vi "optionsAcq_channel_select.vi"(8 "error in (no error)":errorcluster, 9 "channelType_spectrum":T1, 10 "channel DUT (index)":i32, 11 "Thorlabs_OSA300_64 in":refnum<class "OSA300.lvclass">) -> (0 "error out":errorcluster, 2 "channel DUT out":i32, 3 "Thorlabs_OSA300_64 out":refnum<class "OSA300.lvclass">)   [LabVIEW 2010, in "OSA300.lvclass"]
doc: "Models within the OSA300/Redstone series typically have two detection channels, together they provide the total specified wavelength range. The channel index must be selected when acquiring interferograms, the default channel index is zero after init.vi. \n\nWhen acquiring a spectra, either the total wavelength range can be selected, (the ranges provided by all channels stiched together, referred to as a stiched spectra), or the range corresponding to one channel index.\n\nThe wavelength range associated with each channel can be read with instrumentProperties_channels.vi."
uses:
  OSA300.lvclass
  _misc/Thorlabs_FTS_misc.llb/channelType_spectrum.ctl
  OSA20X_misc.lvlib
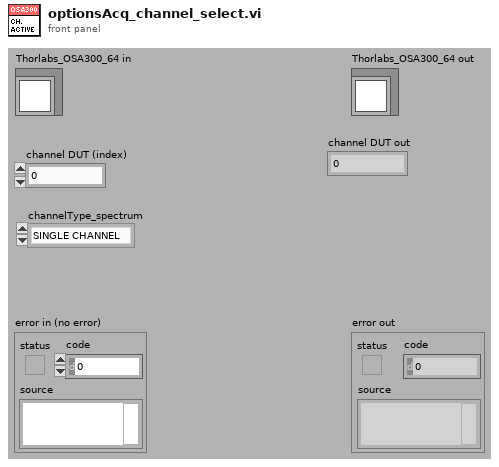
[diagram p1: front panel]
types:
  T1 = typedef "OSA20X_misc.lvlib/channelType_spectrum.ctl" = enum16{"SINGLE CHANNEL", "STICHED"}
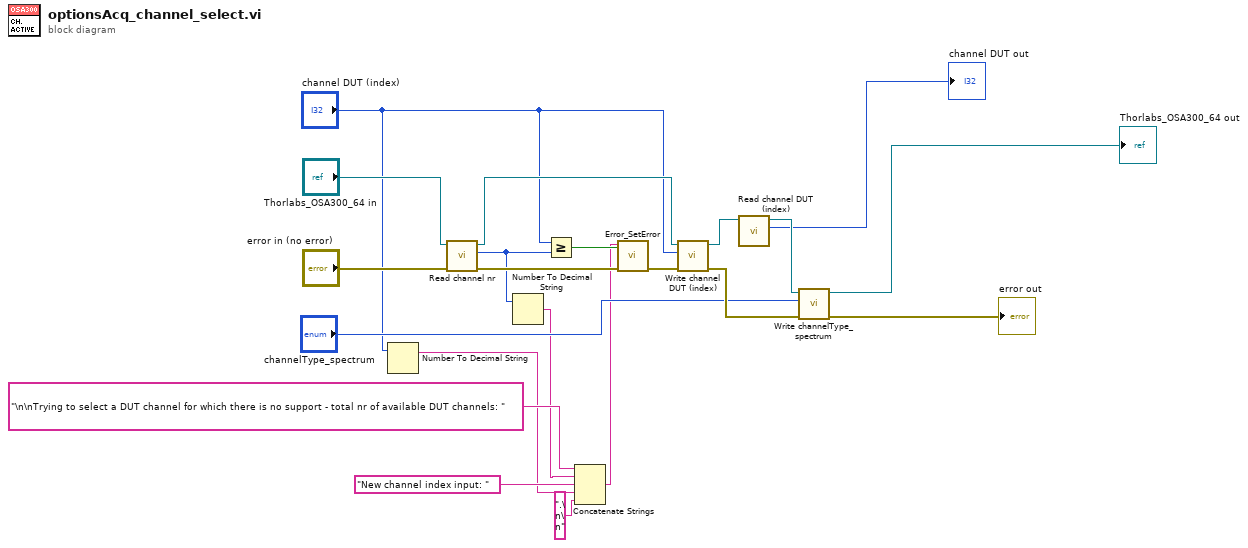
[diagram p0: block diagram]
diagram:
  n1 = Number To Decimal String(number="channel DUT (index)") -> (decimal integer string=w6:string)  [unwired: 1 in]
  n2 = call "Read channel nr.vi"("error in (no error)"="error in (no error)", "OSA300 in"="Thorlabs_OSA300_64 in") -> ("error out"=w14:errorcluster, "channel nr"=w10:i32, "OSA300 out"=w13:refnum<class "OSA300.lvclass">)  [unwired: 7 in]
  n3 = Number To Decimal String(number=w10) -> (decimal integer string=w9:string)  [unwired: 1 in]
  n4 = Greater Or Equal?(x="channel DUT (index)", y=w10) -> (x >= y?=w15:bool)
  n5 = Concatenate Strings("\n\nTrying to select a DUT channel for which there is no support - total nr of available DUT channels: " ("source(\"\")"), w9, "New channel index input: " ("string"), w6, ".\n\n" ("string")) -> (w4:string)
  n6 = call "Error_SetError.vi"("error in"=w14, "status (true)"=w15, "source(\"\")"=w4) -> ("error out"=w12:errorcluster)  [unwired: 4 in]
  n7 = call "Write channel DUT (index).vi"("error in (no error)"=w12, "channel DUT (index)"="channel DUT (index)", "OSA300 in"=w13) -> ("error out"=w21:errorcluster, "OSA300 out"=w3:refnum<class "OSA300.lvclass">)  [unwired: 7 in]
  n8 = call "Read channel DUT (index).vi"("OSA300 in"=w3) -> ("channel ifrgrm (index)"=→"channel DUT out":i32, "OSA300 out"=w2:refnum<class "OSA300.lvclass">)  [unwired: 8 in, 1 out]
  n9 = call "Write channelType_spectrum.vi"("error in (no error)"=w21, "channelType_spectrum"="channelType_spectrum", "OSA300 in"=w2) -> ("error out"=→"error out":errorcluster, "OSA300 out"=→"Thorlabs_OSA300_64 out":refnum<class "OSA300.lvclass">)  [unwired: 7 in]
